vi "MeasGroupResult.vi"(8 "error in (no error)":errorcluster, 10 "measurement_group_id":u16, 11 "ByteGSAPIBase in":refnum<class "ByteGSAPIBase.lvclass">) -> (0 "error out":errorcluster, 1 "measurements":cluster{"id":u32, "passed":bool}[](array[cluster]), 2 "measurement_group_passed":bool, 3 "ByteGSAPIBase out":refnum<class "ByteGSAPIBase.lvclass">)   [LabVIEW 2019, in "ByteGSWebAPI.lvlib" / "ByteGSAPIBase.lvclass"]
uses:
  ByteGSAPIBase.lvclass
  <vilib>/Bytelabs/ByteREST/ByteRESTClass/ByteRESTBase/HTTP/Status_Code.ctl
  TypeDef/Meas_Group_Res_REQ.ctl
  TypeDef/Meas_Group_Res_RESP.ctl
  ByteGSAPIBase.lvclass/ByteGSAPIBase.ctl
  <vilib>/Bytelabs/ByteREST/ByteRESTClass/ByteRESTBase/RESTBase.lvclass
panel:
  # "MeasGroupResult\nendpoint: meas-group-result\n\ntype: POST\n\nrequest body:\n\n\n\n{\n  \"measurement_group_id\": id del gruppo di misure\n}\nresponse body:\n\n\n\n{\n  measurement_group_passed: true/false\n  measurements : [{\n  id:xxxx,passed:true/false,\n  },{\n  id:yyyy,passed:true/false,\n  },{\n  id:zzzz,passed:true/false,\n  },]\n}"
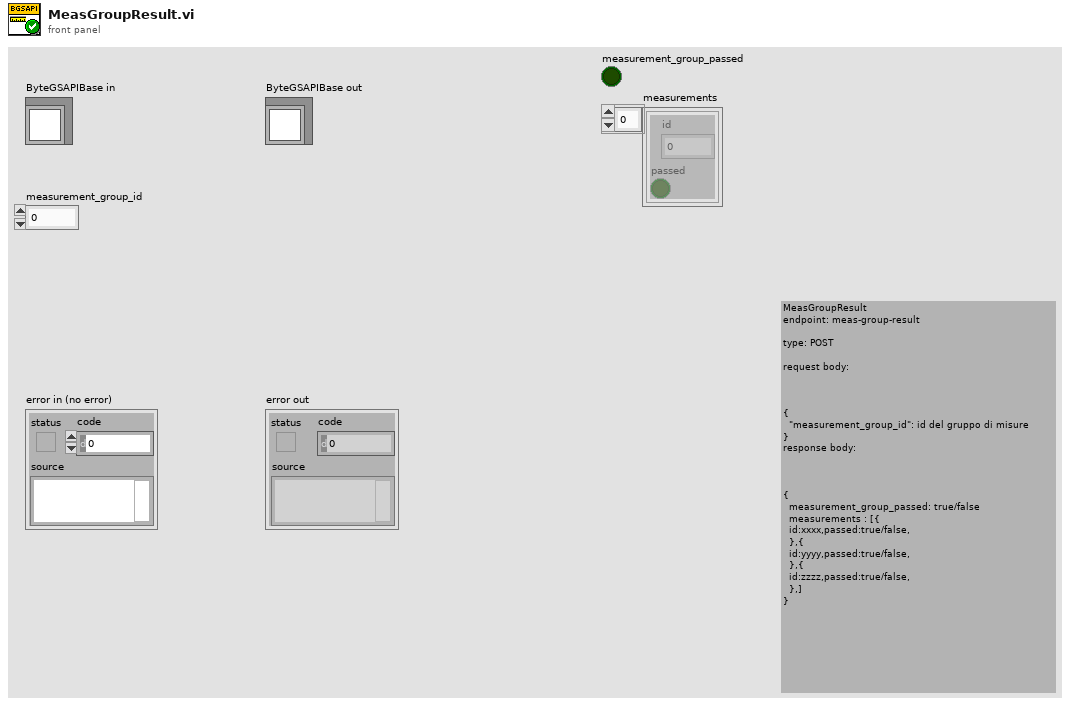
[diagram p1: front panel]
types:
  T1 = typedef "ByteGSWebAPI.lvlib/ByteGSAPIBase.lvclass/Meas_Group_Res_RESP.ctl" = cluster{"measurement_group_passed":bool, "measurements":cluster{"id":u32, "passed":bool}[]}
  T2 = typedef "ByteGSWebAPI.lvlib/ByteGSAPIBase.lvclass/Meas_Group_Res_REQ.ctl" = cluster{"measurement_group_id":u32}
  T3 = typedef "ByteREST.lvlib/RESTBase.lvclass/Status_Code.ctl" = u16
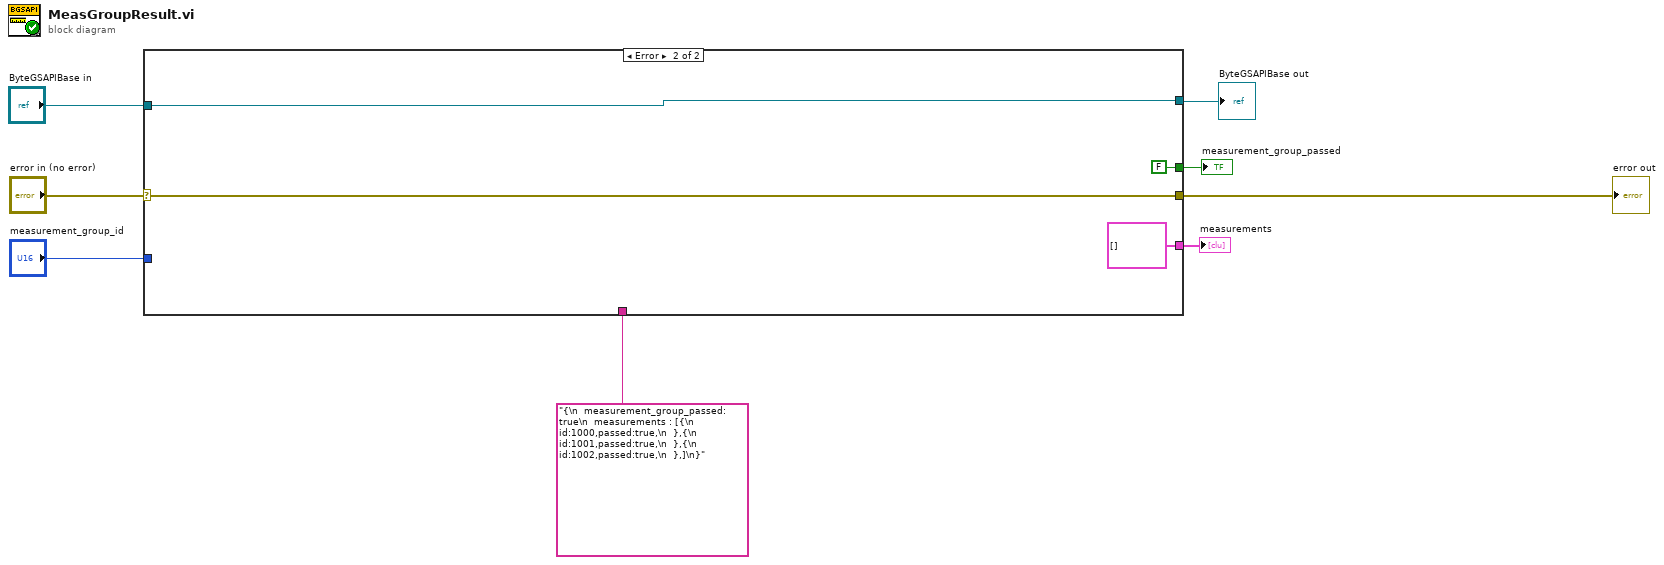
[diagram p0: block diagram]
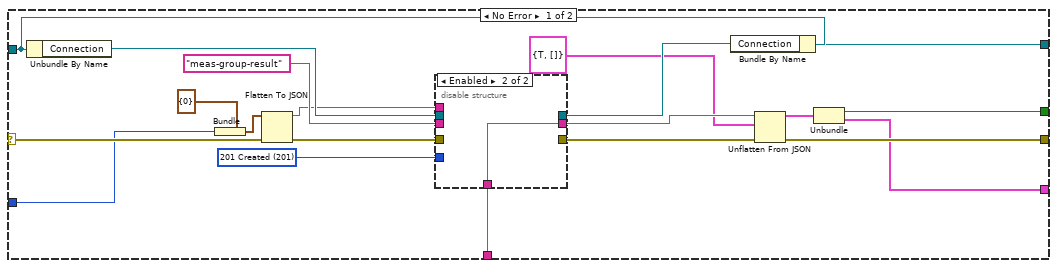
[diagram p2: hidden frame]
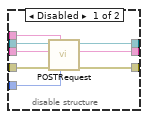
[diagram p3: hidden frame]
diagram:
  n1 = case shown="Error" "error in (no error)" {
    selector: "error in (no error)" -> [w23 w41]
    tunnel: [w17 w41] -> w7
    tunnel: [w26 w40] -> w5
    tunnel: "ByteGSAPIBase in" -> [w28 w40]
    tunnel: "{\n  measurement_group_passed: true\n  measurements : [{\n  id:1000,passed:true,\n  },{\n  id:1001,passed:true,\n  },{\n  id:1002,passed:true,\n  },]\n}" -> [w15 _]
    tunnel: "measurement_group_id" -> [w13 _]
    tunnel: [w10 FALSE ("measurement_group_passed")] -> w2
    tunnel: [w9 cluster{"id":u32, "passed":bool}[] [] ("measurements")] -> w1
    frame No Error {
      w20 = T3 201 items=["200 OK"=200, "201 Created"=201, "400 Bad Request"=400, "401 Unauthorized"=401, "403 Forbidden"=403, "404 Not Found"=404, "405 Method Not Allowed"=405, "406 Not Acceptable"=406, "500 Internal Server Error"=500] ("expected response")
      n2 = Unbundle By Name(w28) -> ("Connection"=w27:refnum<class "RESTBase.lvclass">)
      n3 = Bundle(cluster=T2 {"measurement_group_id"=0} ("MeasGroupResult_REQ"), "measurement_group_id"=w13) -> (w16:T2)
      n4 = Flatten To JSON(anything=w16, error in (no error)=w23) -> (JSON string=w18:string, 11:w19:errorcluster)  [unwired: 1 in]
      n5 = disable-structure shown="Enabled" {
        disable-tunnel: w27 -> [w36 _]
        disable-tunnel: [w35 _] -> w25
        disable-tunnel: "meas-group-result" ("Request") -> [w34 _]
        disable-tunnel: [w33 w37] -> w22
        disable-tunnel: [w32 _] -> w21
        disable-tunnel: w20 -> [w31 _]
        disable-tunnel: w19 -> [w30 _]
        disable-tunnel: w18 -> [w29 _]
        disable-tunnel: w15 -> [_ w37]
        frame Disabled {
          n6 = call-dynamic "POSTRequest.vi"("expected response"=w31, "Body in"=w29, "error in (no error)"=w30, "Request"=w34, "ByteRESTBase in"=w36) -> ("error out"=w32:errorcluster, "Body"=w33:string, "ByteRESTBase out"=w35:refnum<class "RESTBase.lvclass">)  [unwired: 3 in, 1 out]
        }
        frame Enabled {
        }
      }
      n7 = Bundle By Name(cluster=w28, "Connection"=w25) -> (w26:refnum<class "ByteGSAPIBase.lvclass">)
      n8 = Unflatten From JSON(JSON string=w22, type and defaults=T1 {"measurement_group_passed"=TRUE, "measurements"=[]}, error in (no error)=w21) -> (value=w14:T1, error out=w17:errorcluster)  [unwired: 4 in]
      n9 = Unbundle(w14) -> ("measurement_group_passed"=w10:bool, "measurements"=w9:cluster{"id":u32, "passed":bool}[])
    }
    frame Error {
    }
  }
  "error out" <- w7
  "ByteGSAPIBase out" <- w5
  "measurement_group_passed" <- w2
  "measurements" <- w1
